vi "Get_data_within_cursors.vi"(10 "Cursors":dbl[](array[numeric]), 11 "Waveform Data":waveform(dbl)) -> (3 "waveform out":waveform(dbl))   [LabVIEW 2015]
uses:
  <vilib>/Waveform/WDTOps.llb/WDT Get Waveform Subset DBL.vi
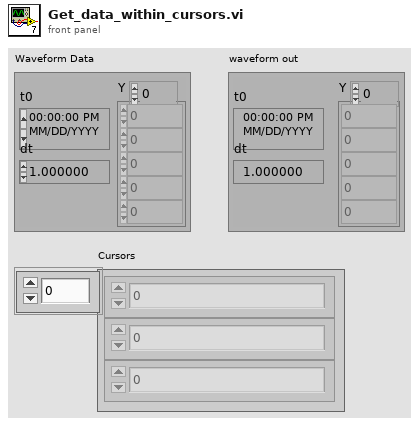
[diagram p1: front panel]
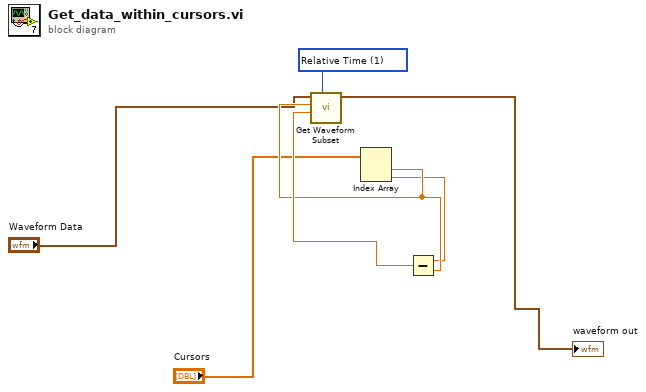
[diagram p0: block diagram]
diagram:
  w6 = u16 1 items=["Samples", "Relative Time"] ("start/duration format")
  n1 = Index Array(array="Cursors") -> (element #1=w4:dbl, element #2=w3:dbl)  [unwired: 2 in]
  n2 = Subtract(x=w3, y=w4) -> (x-y=w5:dbl)
  n3 = call-poly <vilib>:"Get Waveform Subset.vi"("start/duration format"=w6, "duration"=w5, "start samples/time"=w4, "waveform in"="Waveform Data") -> ("waveform out"=→"waveform out":waveform(dbl))  [unwired: 2 in, 3 out]
